vi "Manual Test.vi"() -> ()   [LabVIEW 2020, in "driver_flodx_rtd.lvlib"]
doc: "Manually test all functions and commands of device"
uses:
  <instrlib>/RxnRover/FloDx RTD Driver/driver_flodx_rtd.lvlib
panel:
  in  "Set Verbose Mode":bool
  in  "Verbose Mode":sgl
  in  "Get Standy Mode":bool
  in  "Set Standby Mode":bool
  out "Standby Mode?":dbl
  in  "Standby Mode":sgl
  in  "Get Mode":bool
  in  "Set Mode":bool
  in  "Mode 0(sense) 1(Heat) 2(Cool)":sgl
  out "Mode":dbl
  in  "Get Temperature":bool
  out "Temperature":dbl
  in  "Get Kp":bool
  in  "Get Ki":bool
  in  "Get Kd":bool
  out "Kd":dbl
  out "Kp":dbl
  out "Ki":dbl
  in  "Set Kd":bool
  in  "Set Kp":bool
  in  "Set Ki":bool
  in  "SetKd":dbl
  in  "SetKp":dbl
  in  "SetKi":dbl
  in  "Get Set Point":bool
  in  "Get Set Point Min":bool
  in  "Get Set Point Max":bool
  in  "Set Point Max":bool
  in  "Set Point Min":bool
  in  "Set Point":bool
  out "Set Point Max":dbl
  in  "SetPointMax":dbl
  out "Set Point Min":dbl
  in  "SetPointMin":dbl
  out "Set Point":dbl
  in  "SetPoint":dbl
  in  "Set Address":sgl
  out "Address":dbl
  in  "Print Address":bool
  in  "Set Address":bool
  out "Raw Response":string
  in  "Exit Config":bool
  in  "(1)Save (0)Reverts":sgl
  out "(1)Saved (0)Reverted":dbl
  in  "Enter CONFIG State":bool
  in  "Print Device Type":bool
  out "ConfigState":bool
  out "Device Type":dbl
  in  "Address":u8
  in  "error in":errorcluster
  in  "VISA resource name":refnum<visa-resource-name>
  out "error out":errorcluster
  out "VISA resource name out":refnum<visa-resource-name>
  in  "Close Communication with Device":bool
  in  "Initialize  For Test DO THIS BEFORE RUNNING ANY TESTS":bool
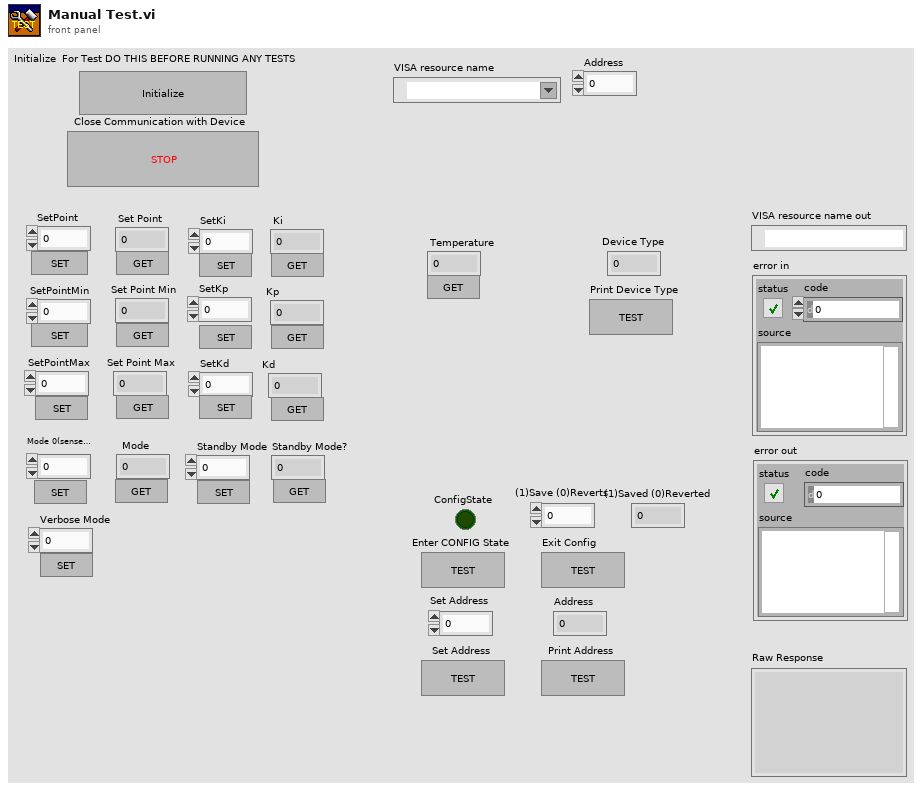
[diagram p1: front panel]
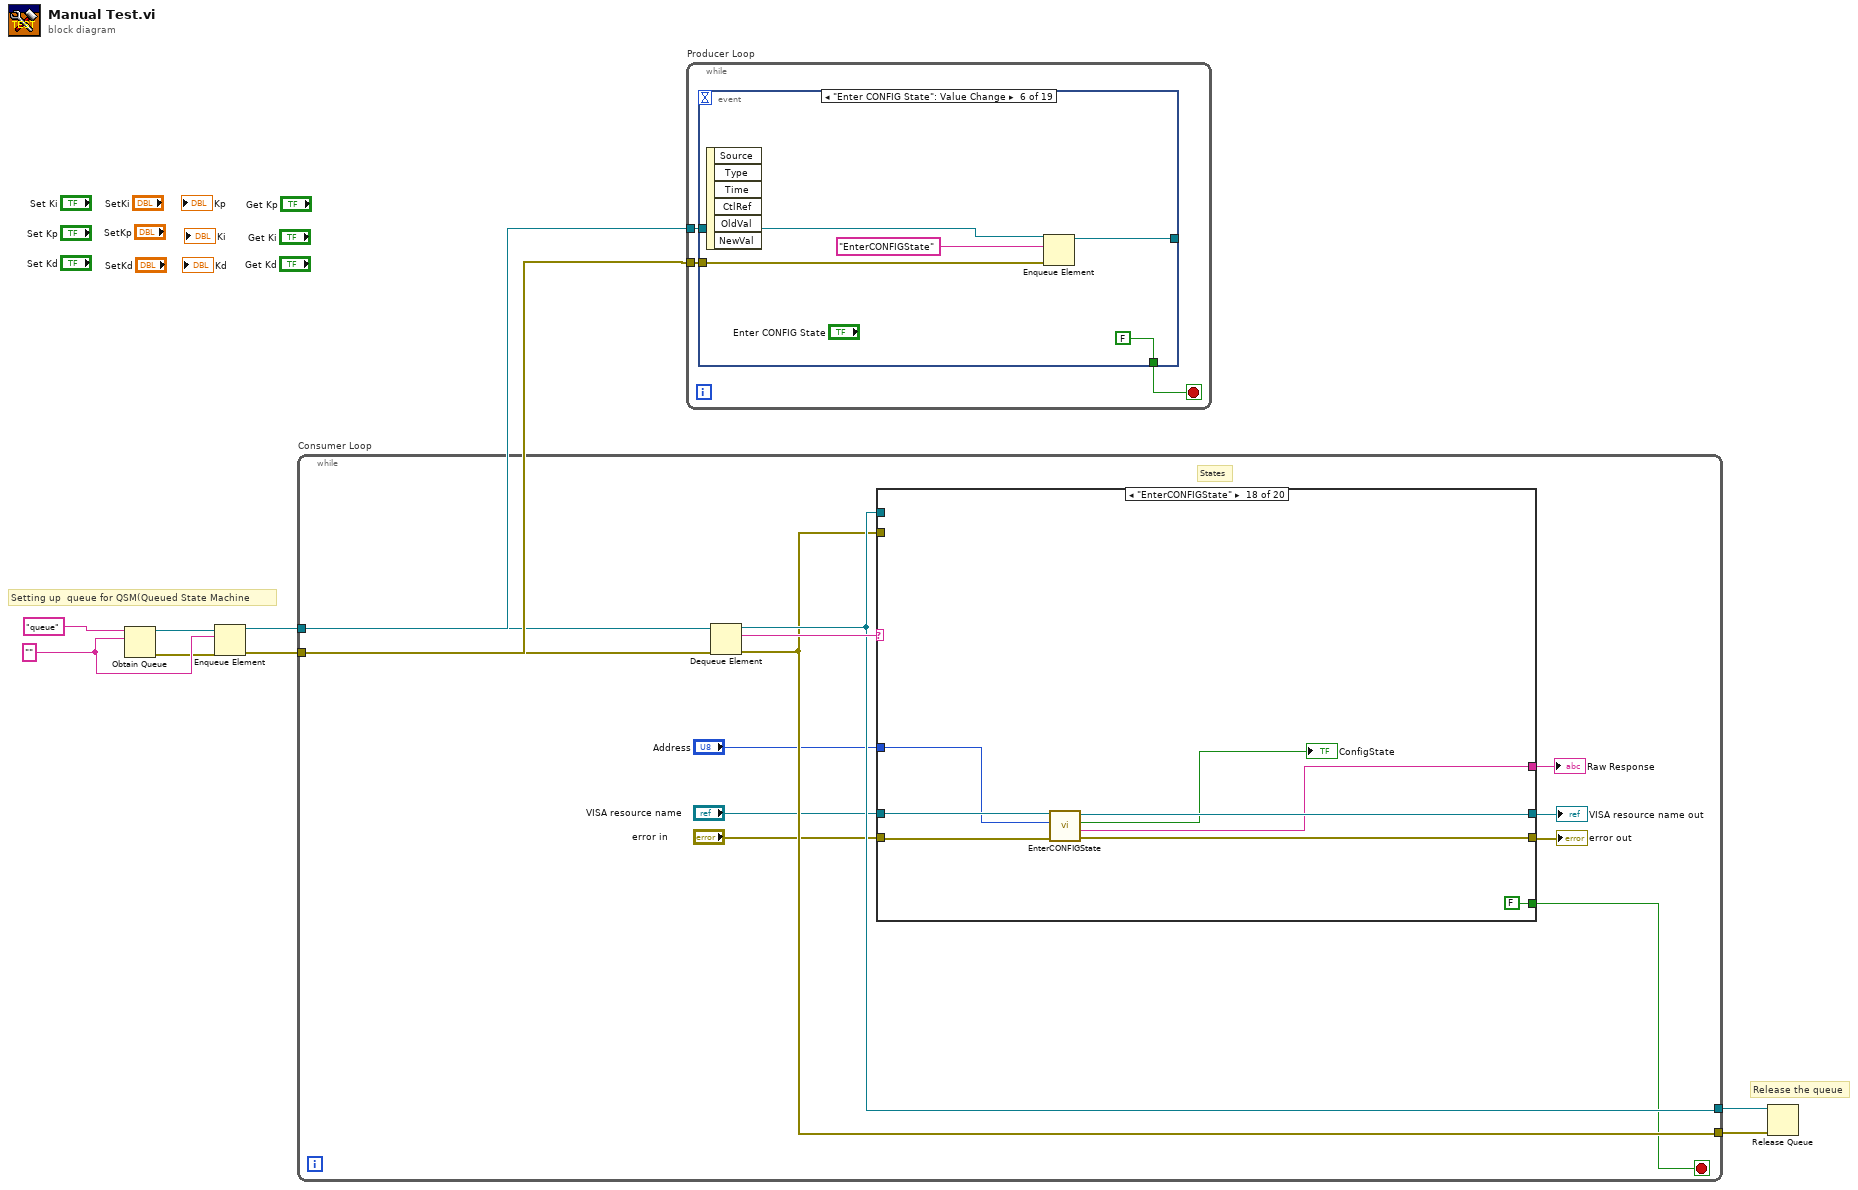
[diagram p0: block diagram]
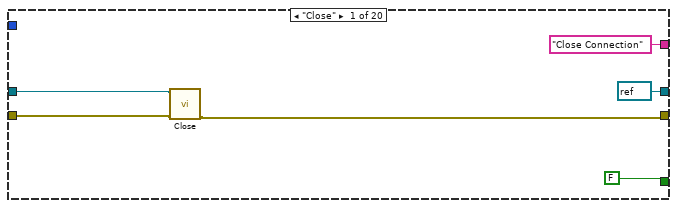
[diagram p2: hidden frame]
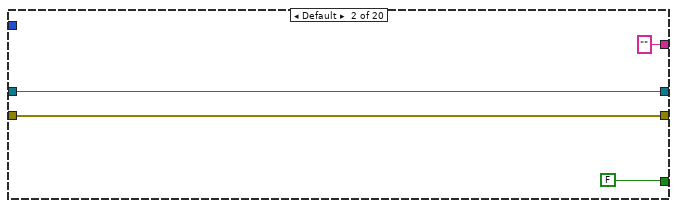
[diagram p3: hidden frame]
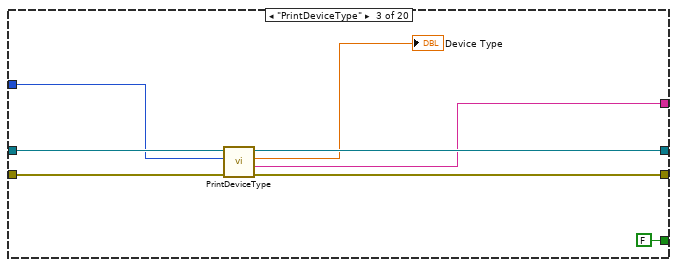
[diagram p4: hidden frame]
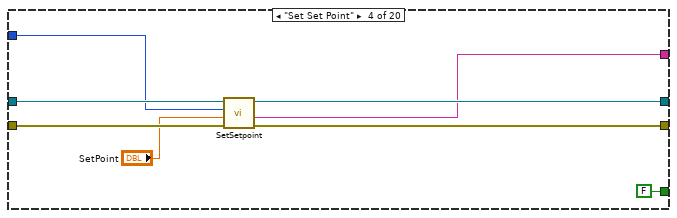
[diagram p5: hidden frame]
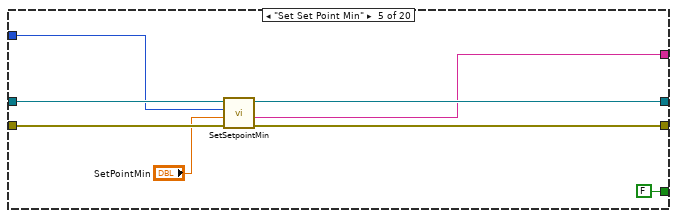
[diagram p6: hidden frame]
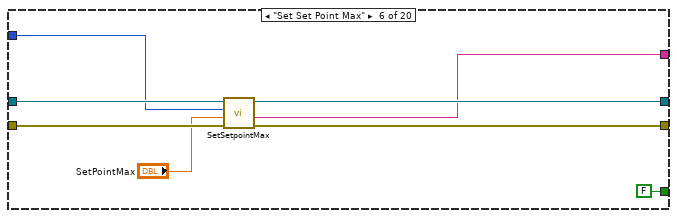
[diagram p7: hidden frame]
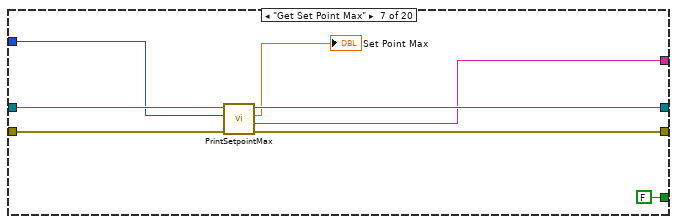
[diagram p8: hidden frame]
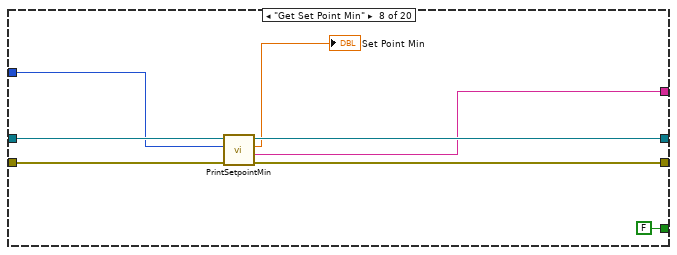
[diagram p9: hidden frame]
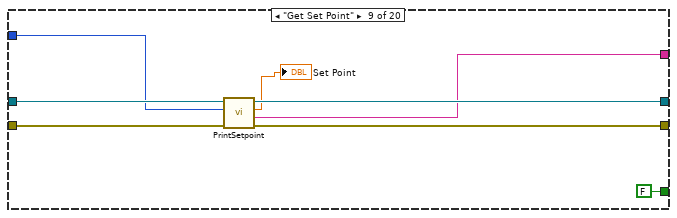
[diagram p10: hidden frame]
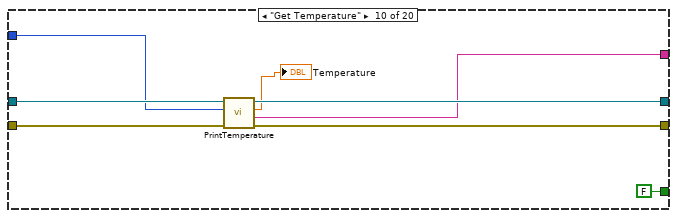
[diagram p11: hidden frame]
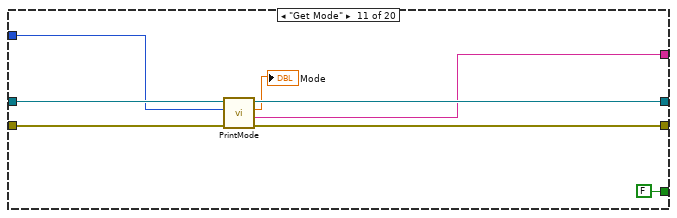
[diagram p12: hidden frame]
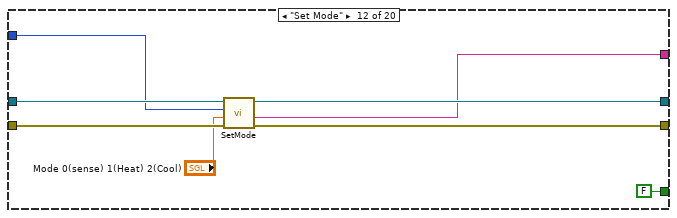
[diagram p13: hidden frame]
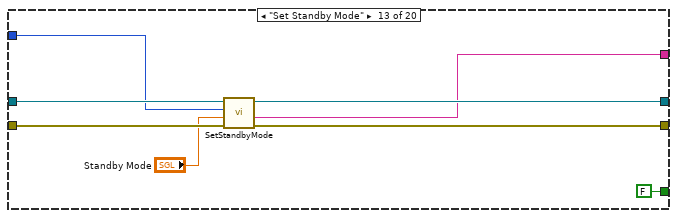
[diagram p14: hidden frame]
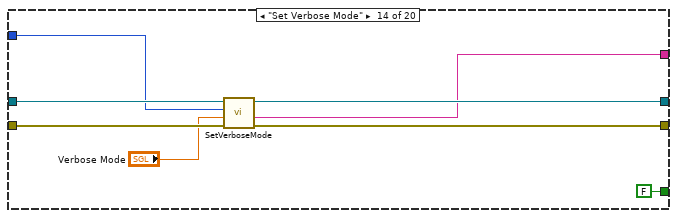
[diagram p15: hidden frame]
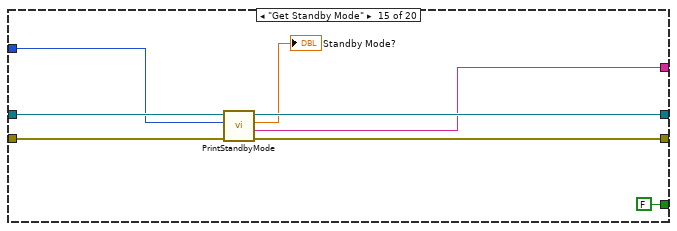
[diagram p16: hidden frame]
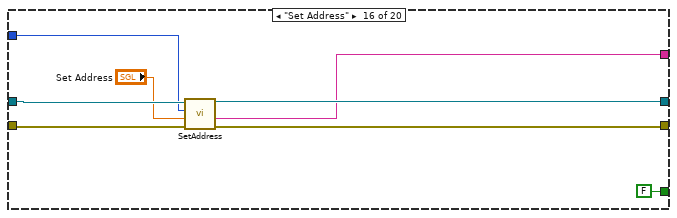
[diagram p17: hidden frame]
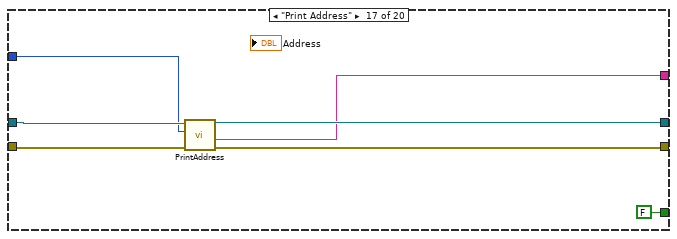
[diagram p18: hidden frame]
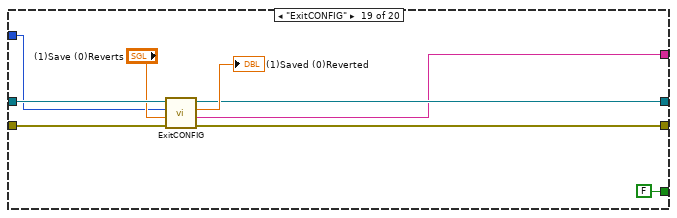
[diagram p19: hidden frame]
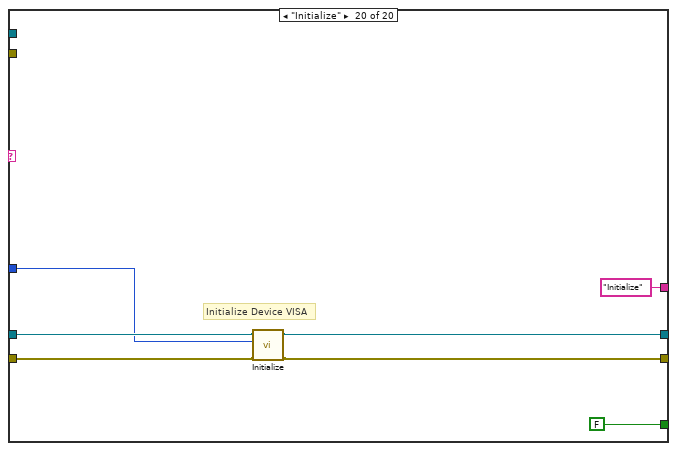
[diagram p20: hidden frame]
diagram:
  w7 = ""
  # "Release the queue"
  # "Setting up  queue for QSM(Queued State Machine"
  n1 = Obtain Queue(name (unnamed)="queue", element data type=w7) -> (queue out=w6:refnum<queue>, error out=w5:errorcluster)  [unwired: 3 in, 1 out]
  n2 = Enqueue Element(queue=w6, element=w7, error in (no error)=w5) -> (queue out=w1:refnum<queue>, error out=w2:errorcluster)  [unwired: 1 in, 1 out]
  n3 = while "Consumer Loop" {
    tunnel: [w17] -> w4
    tunnel: [w16] -> w3
    tunnel: w2 -> [w20]
    tunnel: w1 -> [w19]
    stop <- w11 stop-if-true
    # "States"
    n4 = Dequeue Element(queue=w19, error in (no error)=w20) -> (queue out=w17:refnum<queue>, element=w18:string, error out=w16:errorcluster)  [unwired: 1 in, 1 out]
    n5 = case shown="\"EnterCONFIGState\"" w18 {
      tunnel: w17 -> [_ _ _ _ _ _ _ _ _ _ _ _ _ _ _ _ _ _ _ _]
      tunnel: w16 -> [_ _ _ _ _ _ _ _ _ _ _ _ _ _ _ _ _ _ _ _]
      tunnel: "VISA resource name" -> [w22 w30 w35 w44 w52 w60 w68 w76 w84 w92 w100 w108 w116 w124 w132 w142 w149 w154 w163 w172]
      tunnel: "error in" -> [w23 w29 w34 w43 w51 w59 w67 w75 w83 w91 w99 w107 w115 w123 w131 w135 w143 w155 w162 w169]
      tunnel: [refnum<visa-resource-name> refnum ("VISA resource name out") w30 w37 w45 w53 w61 w69 w77 w85 w93 w101 w109 w117 w125 w133 w140 w147 w157 w164 w171] -> w13
      tunnel: [w24 w29 w38 w46 w54 w62 w70 w78 w86 w94 w102 w110 w118 w126 w134 w141 w148 w156 w165 w170] -> w12
      tunnel: [FALSE FALSE FALSE FALSE FALSE FALSE FALSE FALSE FALSE FALSE FALSE FALSE FALSE FALSE FALSE FALSE FALSE FALSE FALSE FALSE] -> w11
      tunnel: "Address" -> [_ _ w33 w42 w50 w58 w66 w74 w82 w90 w98 w106 w114 w122 w130 w136 w144 w153 w160 w167]
      tunnel: ["Close Connection" ("Raw Response") "" ("Raw Response") w31 w40 w48 w56 w64 w72 w80 w88 w96 w104 w112 w120 w128 w138 w145 w150 w158 "Initialize" ("Raw Response")] -> w10
      frame "Close" {
        n6 = call <instrlib>:"Close.vi"("error in (no error)"=w23, "VISA resource name"=w22) -> ("error out"=w24:errorcluster)  [unwired: 9 in]
      }
      frame Default {
      }
      frame "PrintDeviceType" {
        n7 = call <instrlib>:"PrintDeviceType.vi"("error in (no error)"=w34, "Address"=w33, "VISA resource name"=w35) -> ("error out"=w38:errorcluster, "Raw Response"=w31:string, "Device Type"=→"Device Type":dbl, "VISA resource name out"=w37:refnum<visa-resource-name>)  [unwired: 5 in]
      }
      frame "Set Set Point" {
        n8 = call <instrlib>:"SetSetpoint.vi"("error in (no error)"=w43, "Setpoint (C)"="SetPoint", "Address"=w42, "VISA resource name"=w44) -> ("error out"=w46:errorcluster, "Raw Response"=w40:string, "VISA resource name out"=w45:refnum<visa-resource-name>)  [unwired: 5 in]
      }
      frame "Set Set Point Min" {
        n9 = call <instrlib>:"SetSetpointMin.vi"("error in (no error)"=w51, "Setpoint Min (C)"="SetPointMin", "Address"=w50, "VISA resource name"=w52) -> ("error out"=w54:errorcluster, "Raw Response"=w48:string, "VISA resource name out"=w53:refnum<visa-resource-name>)  [unwired: 5 in]
      }
      frame "Set Set Point Max" {
        n10 = call <instrlib>:"SetSetpointMax.vi"("error in (no error)"=w59, "Setpoint Max (C)"="SetPointMax", "Address"=w58, "VISA resource name"=w60) -> ("error out"=w62:errorcluster, "Raw Response"=w56:string, "VISA resource name out"=w61:refnum<visa-resource-name>)  [unwired: 5 in]
      }
      frame "Get Set Point Max" {
        n11 = call <instrlib>:"PrintSetpointMax.vi"("error in (no error)"=w67, "Address"=w66, "VISA resource name"=w68) -> ("error out"=w70:errorcluster, "Raw Response"=w64:string, "Max SetPoint (C)"=→"Set Point Max":dbl, "VISA resource name out"=w69:refnum<visa-resource-name>)  [unwired: 5 in]
      }
      frame "Get Set Point Min" {
        n12 = call <instrlib>:"PrintSetpointMin.vi"("error in (no error)"=w75, "Address"=w74, "VISA resource name"=w76) -> ("error out"=w78:errorcluster, "Raw Response"=w72:string, "Min SetPoint (C)"=→"Set Point Min":dbl, "VISA resource name out"=w77:refnum<visa-resource-name>)  [unwired: 5 in]
      }
      frame "Get Set Point" {
        n13 = call <instrlib>:"PrintSetpoint.vi"("error in (no error)"=w83, "Address"=w82, "VISA resource name"=w84) -> ("error out"=w86:errorcluster, "Raw Response"=w80:string, "SetPoint (C)"=→"Set Point":dbl, "VISA resource name out"=w85:refnum<visa-resource-name>)  [unwired: 5 in]
      }
      frame "Get Temperature" {
        n14 = call <instrlib>:"PrintTemperature.vi"("error in (no error)"=w91, "Address"=w90, "VISA resource name"=w92) -> ("error out"=w94:errorcluster, "Raw Response"=w88:string, "Temperature"=→"Temperature":dbl, "VISA resource name out"=w93:refnum<visa-resource-name>)  [unwired: 5 in]
      }
      frame "Get Mode" {
        n15 = call <instrlib>:"PrintMode.vi"("error in (no error)"=w99, "Address"=w98, "VISA resource name"=w100) -> ("error out"=w102:errorcluster, "Raw Response"=w96:string, "Mode 0(sense) 1(Heat) 2(Cool)"=→"Mode":dbl, "VISA resource name out"=w101:refnum<visa-resource-name>)  [unwired: 5 in]
      }
      frame "Set Mode" {
        n16 = call <instrlib>:"SetMode.vi"("error in (no error)"=w107, "Mode 0(sense) 1(Heat) 2(Cool)"="Mode 0(sense) 1(Heat) 2(Cool)", "Address"=w106, "VISA resource name"=w108) -> ("error out"=w110:errorcluster, "Raw Response"=w104:string, "VISA resource name out"=w109:refnum<visa-resource-name>)  [unwired: 5 in]
      }
      frame "Set Standby Mode" {
        n17 = call <instrlib>:"SetStandbyMode.vi"("error in (no error)"=w115, "Standby Mode"="Standby Mode", "Address"=w114, "VISA resource name"=w116) -> ("error out"=w118:errorcluster, "Raw Response"=w112:string, "VISA resource name out"=w117:refnum<visa-resource-name>)  [unwired: 5 in]
      }
      frame "Set Verbose Mode" {
        n18 = call <instrlib>:"SetVerboseMode.vi"("error in (no error)"=w123, "Verbose Mode"="Verbose Mode", "Address"=w122, "VISA resource name"=w124) -> ("error out"=w126:errorcluster, "Raw Response"=w120:string, "VISA resource name out"=w125:refnum<visa-resource-name>)  [unwired: 5 in]
      }
      frame "Get Standby Mode" {
        n19 = call <instrlib>:"PrintStandbyMode.vi"("error in (no error)"=w131, "Address"=w130, "VISA resource name"=w132) -> ("error out"=w134:errorcluster, "Raw Response"=w128:string, "Stanby Mode?"=→"Standby Mode?":dbl, "VISA resource name out"=w133:refnum<visa-resource-name>)  [unwired: 5 in]
      }
      frame "Set Address" {
        n20 = call <instrlib>:"SetAddress.vi"("error in (no error)"=w135, "Address(New)"="Set Address", "Address(Current)"=w136, "VISA resource name"=w142) -> ("error out"=w141:errorcluster, "Raw Response"=w138:string, "VISA resource name out"=w140:refnum<visa-resource-name>)  [unwired: 5 in]
      }
      frame "Print Address" {
        n21 = call <instrlib>:"PrintAddress.vi"("error in (no error)"=w143, "Address"=w144, "VISA resource name"=w149) -> ("error out"=w148:errorcluster, "Raw Response"=w145:string, "VISA resource name out"=w147:refnum<visa-resource-name>)  [unwired: 6 in]
      }
      frame "EnterCONFIGState" {
        n22 = call <instrlib>:"EnterCONFIGState.vi"("error in (no error)"=w155, "Address"=w153, "VISA resource name"=w154) -> ("error out"=w156:errorcluster, "Raw Response"=w150:string, "ConfigState"=→"ConfigState":bool, "VISA resource name out"=w157:refnum<visa-resource-name>)  [unwired: 5 in]
      }
      frame "ExitCONFIG" {
        n23 = call <instrlib>:"ExitCONFIG.vi"("error in (no error)"=w162, "(1)Save (0)Reverts"="(1)Save (0)Reverts", "Address"=w160, "VISA resource name"=w163) -> ("error out"=w165:errorcluster, "Raw Response"=w158:string, "(1)Saved (0)Reverted"=→"(1)Saved (0)Reverted":dbl, "VISA resource name out"=w164:refnum<visa-resource-name>)  [unwired: 4 in]
      }
      frame "Initialize" {
        # "Initialize Device VISA"
        n24 = call <instrlib>:"Initialize.vi"("error in (no error)"=w169, "Address"=w167, "VISA resource name"=w172) -> ("error out"=w170:errorcluster, "VISA resource name out"=w171:refnum<visa-resource-name>)  [unwired: 6 in, 1 out]
      }
    }
    "error out" <- w12
    "VISA resource name out" <- w13
    "Raw Response" <- w10
  }
  n25 = while "Producer Loop" {
    tunnel: w2 -> [w176]
    tunnel: w1 -> [w175]
    stop <- w174 stop-if-true
    n26 = event shown="[5] \"Enter CONFIG State\": Value Change" {
      selector: _ -> [_ _ _ _ _ _ _ _ _ _ _ _ _ _ _ _ _ _ _]
      dyn-events: _ -> [_ _ _ _ _ _ _ _ _ _ _ _ _ _ _ _ _ _ _]
      timeout: _ -> [_ _ _ _ _ _ _ _ _ _ _ _ _ _ _ _ _ _ _]
      tunnel: w176 -> [w180 w185 w190 w195 w200 w205 w210 w215 w220 w225 w230 w235 w240 w245 w250 w255 w260 w265 w270]
      tunnel: w175 -> [w179 w184 w189 w194 w199 w204 w209 w214 w219 w224 w229 w234 w239 w244 w249 w254 w259 w264 w269]
      tunnel: [w178 w183 w188 w193 w198 w203 w208 w213 w218 w223 w228 w233 w238 w243 w248 w253 w258 w263 w268] -> _
      tunnel: [FALSE FALSE FALSE FALSE FALSE FALSE FALSE FALSE FALSE FALSE FALSE FALSE FALSE FALSE FALSE FALSE FALSE FALSE FALSE] -> w174
      event "Initialize  For Test DO THIS BEFORE RUNNING ANY TESTS": Value Change {
        n27 = event-data() -> ()  [unwired: 1 in, 6 out]
        n28 = Enqueue Element(queue=w179, element="Initialize", error in (no error)=w180) -> (queue out=w178:refnum<queue>)  [unwired: 1 in, 2 out]
      }
      event "Close Communication with Device": Value Change {
        n29 = event-data() -> ()  [unwired: 1 in, 6 out]
        n30 = Enqueue Element(queue=w184, element="Close", error in (no error)=w185) -> (queue out=w183:refnum<queue>)  [unwired: 1 in, 2 out]
      }
      event "Print Address": Value Change {
        n31 = event-data() -> ()  [unwired: 1 in, 6 out]
        n32 = Enqueue Element(queue=w189, element="Print Address", error in (no error)=w190) -> (queue out=w188:refnum<queue>)  [unwired: 1 in, 2 out]
      }
      event "Set Address": Value Change {
        n33 = event-data() -> ()  [unwired: 1 in, 6 out]
        n34 = Enqueue Element(queue=w194, element="Set Address", error in (no error)=w195) -> (queue out=w193:refnum<queue>)  [unwired: 1 in, 2 out]
      }
      event "Exit Config": Value Change {
        n35 = event-data() -> ()  [unwired: 1 in, 6 out]
        n36 = Enqueue Element(queue=w199, element="ExitCONFIG", error in (no error)=w200) -> (queue out=w198:refnum<queue>)  [unwired: 1 in, 2 out]
      }
      event "Enter CONFIG State": Value Change {
        n37 = event-data() -> ()  [unwired: 1 in, 6 out]
        n38 = Enqueue Element(queue=w204, element="EnterCONFIGState", error in (no error)=w205) -> (queue out=w203:refnum<queue>)  [unwired: 1 in, 2 out]
      }
      event "Print Device Type": Value Change {
        n39 = event-data() -> ()  [unwired: 1 in, 6 out]
        n40 = Enqueue Element(queue=w209, element="PrintDeviceType", error in (no error)=w210) -> (queue out=w208:refnum<queue>)  [unwired: 1 in, 2 out]
      }
      event "Set Point": Value Change {
        n41 = event-data() -> ()  [unwired: 1 in, 6 out]
        n42 = Enqueue Element(queue=w214, element="Set Set Point", error in (no error)=w215) -> (queue out=w213:refnum<queue>)  [unwired: 1 in, 2 out]
      }
      event "Set Point Min": Value Change {
        n43 = event-data() -> ()  [unwired: 1 in, 6 out]
        n44 = Enqueue Element(queue=w219, element="Set Set Point Min", error in (no error)=w220) -> (queue out=w218:refnum<queue>)  [unwired: 1 in, 2 out]
      }
      event "Set Point Max": Value Change {
        n45 = event-data() -> ()  [unwired: 1 in, 6 out]
        n46 = Enqueue Element(queue=w224, element="Set Set Point Max", error in (no error)=w225) -> (queue out=w223:refnum<queue>)  [unwired: 1 in, 2 out]
      }
      event "Get Set Point": Value Change {
        n47 = event-data() -> ()  [unwired: 1 in, 6 out]
        n48 = Enqueue Element(queue=w229, element="Get Set Point", error in (no error)=w230) -> (queue out=w228:refnum<queue>)  [unwired: 1 in, 2 out]
      }
      event "Get Set Point Min": Value Change {
        n49 = event-data() -> ()  [unwired: 1 in, 6 out]
        n50 = Enqueue Element(queue=w234, element="Get Set Point Min", error in (no error)=w235) -> (queue out=w233:refnum<queue>)  [unwired: 1 in, 2 out]
      }
      event "Get Set Point Max": Value Change {
        n51 = event-data() -> ()  [unwired: 1 in, 6 out]
        n52 = Enqueue Element(queue=w239, element="Get Set Point Max", error in (no error)=w240) -> (queue out=w238:refnum<queue>)  [unwired: 1 in, 2 out]
      }
      event "Get Temperature": Value Change {
        n53 = event-data() -> ()  [unwired: 1 in, 6 out]
        n54 = Enqueue Element(queue=w244, element="Get Temperature", error in (no error)=w245) -> (queue out=w243:refnum<queue>)  [unwired: 1 in, 2 out]
      }
      event "Set Mode": Value Change {
        n55 = event-data() -> ()  [unwired: 1 in, 6 out]
        n56 = Enqueue Element(queue=w249, element="Set Mode", error in (no error)=w250) -> (queue out=w248:refnum<queue>)  [unwired: 1 in, 2 out]
      }
      event "Set Standby Mode": Value Change {
        n57 = event-data() -> ()  [unwired: 1 in, 6 out]
        n58 = Enqueue Element(queue=w254, element="Set Standby Mode", error in (no error)=w255) -> (queue out=w253:refnum<queue>)  [unwired: 1 in, 2 out]
      }
      event "Get Standy Mode": Value Change {
        n59 = event-data() -> ()  [unwired: 1 in, 6 out]
        n60 = Enqueue Element(queue=w259, element="Get Standby Mode", error in (no error)=w260) -> (queue out=w258:refnum<queue>)  [unwired: 1 in, 2 out]
      }
      event "Set Verbose Mode": Value Change {
        n61 = event-data() -> ()  [unwired: 1 in, 6 out]
        n62 = Enqueue Element(queue=w264, element="Set Verbose Mode", error in (no error)=w265) -> (queue out=w263:refnum<queue>)  [unwired: 1 in, 2 out]
      }
      event "Get Mode": Value Change {
        n63 = event-data() -> ()  [unwired: 1 in, 6 out]
        n64 = Enqueue Element(queue=w269, element="Get Mode", error in (no error)=w270) -> (queue out=w268:refnum<queue>)  [unwired: 1 in, 2 out]
      }
    }
  }
  n65 = Release Queue(queue=w4, error in (no error)=w3) -> ()  [unwired: 1 in, 3 out]
